vi "LoadTSConfigFile.vi"(0 "Sequence path":path=path "C:/ModisEdge/Scanner/Test Sequence/ModisEdgeScanner.ini", 5 "file name":string="ModisEdgeScanner.ini", 11 "error in (no error)":errorcluster) -> (2 "PS1_COMPort":string, 3 "InterlockDevice":string="Dev6", 4 "SnapOnTestScriptFile":string="G16_PD_TS_v3__G16_OC_TS_v2.txt", 6 "UUT_COMPort":string, 8 "DMM_COMPort":string, 10 "ResultsFolder":string="C:\\temp\\", 13 "PS2_COMPort":string, 14 "DAQDevice":string="Dev4", 15 "error out":errorcluster)   [LabVIEW 2015]
doc: "Use this template to build a VI to use as a subVI."
uses:
  <vilib>/Utility/config.llb/Read Key (String).vi
  <vilib>/Utility/config.llb/NI_LVConfig.lvlib
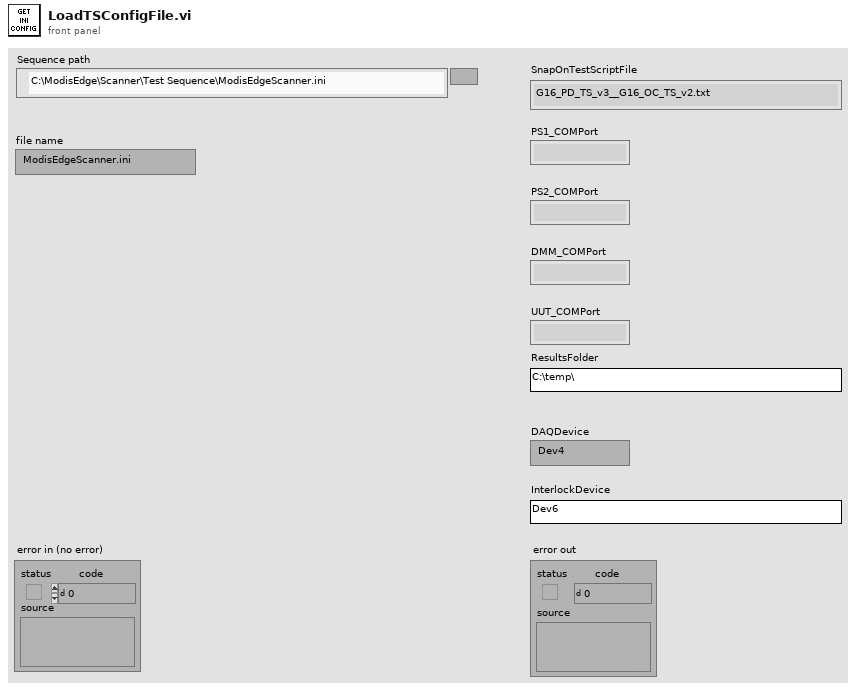
[diagram p1: front panel]
types:
  T1 = typedef "NI_LVConfig.lvlib/Config Data RefNum.ctl" = refnum<k1>
  T2 = typedef "Resource Data.ctl" = cluster{"Resource":string, "Serial Number":string, "Model":string}
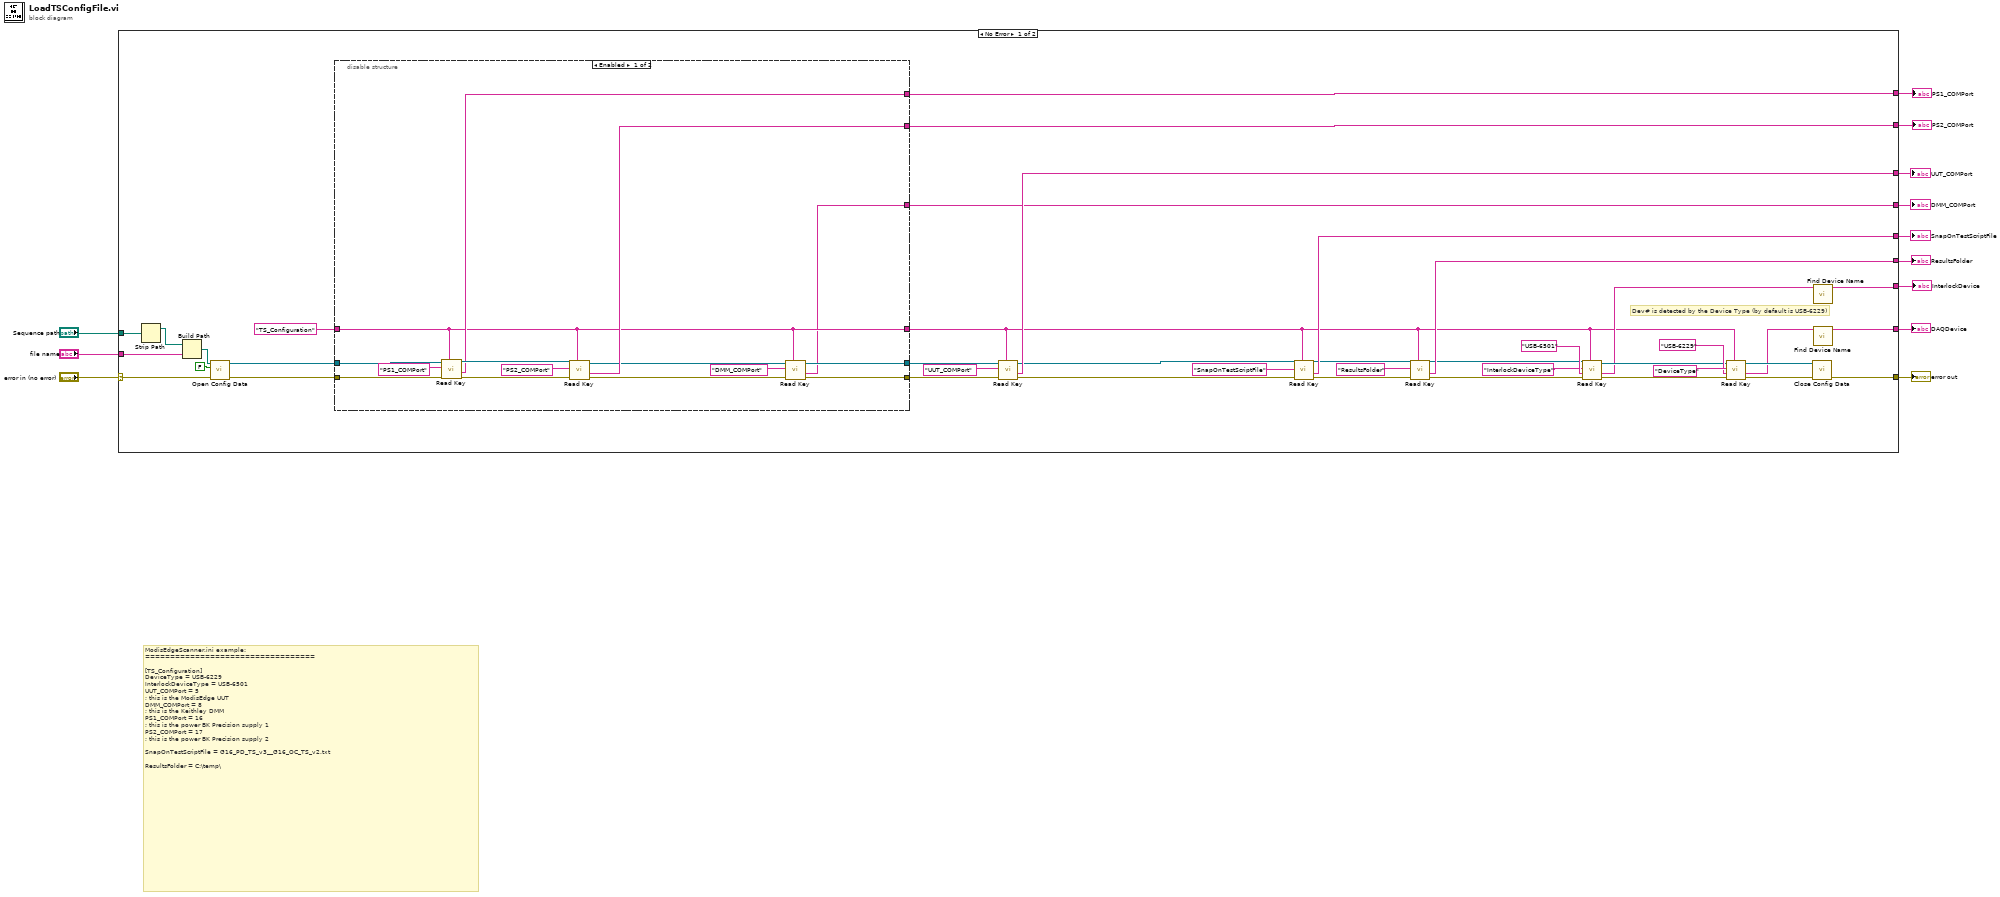
[diagram p0: block diagram]
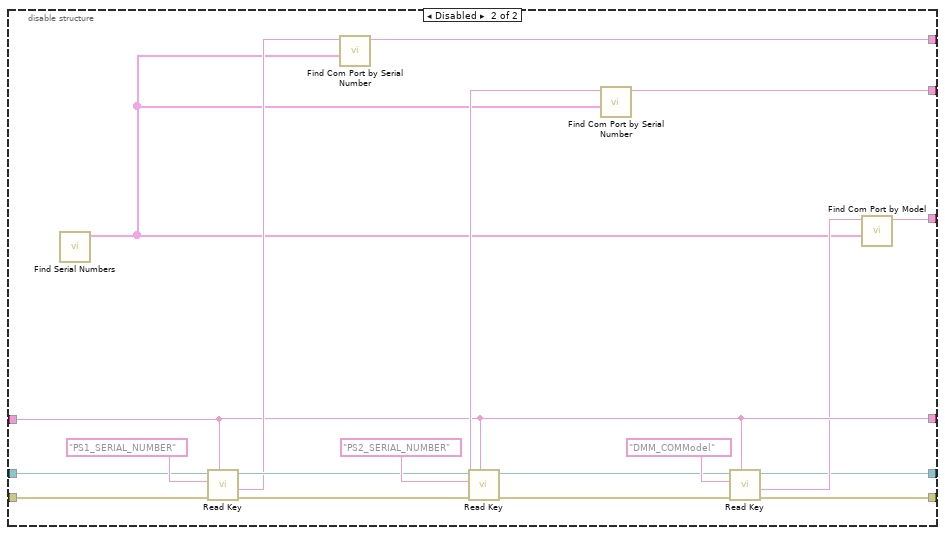
[diagram p2: hidden frame]
diagram:
  # "ModisEdgeScanner.ini example:\n==================================\n\n[TS_Configuration]\nDeviceType = USB-6229\nInterlockDeviceType = USB-6501\nUUT_COMPort = 5 \t\n; this is the ModisEdge UUT\nDMM_COMPort = 8\t\t\n; this is the Keithley DMM\nPS1_COMPort = 16\t\n; this is the power BK Precision supply 1 \nPS2_COMPort = 17\n; this is the power BK Precision supply 2\n\nSnapOnTestScriptFile = G16_PD_TS_v3__G16_OC_TS_v2.txt\n\nResultsFolder = C:\\temp\\"
  n1 = case shown="No Error" "error in (no error)" {
    selector: "error in (no error)" -> [w49 w87]
    tunnel: [w47 w87] -> w11
    tunnel: [w50 _] -> w10
    tunnel: [w48 _] -> w9
    tunnel: [w43 _] -> w8
    tunnel: "Sequence path" -> [w41 _]
    tunnel: [w35 _] -> w7
    tunnel: [w27 _] -> w6
    tunnel: [w16 _] -> w5
    tunnel: "file name" -> [w25 _]
    tunnel: [w22 _] -> w2
    tunnel: [w21 _] -> w1
    frame No Error {
      # "Dev# is detected by the Device Type (by default is USB-6229)"
      n2 = Strip Path(path=w41) -> (stripped path=w26:path)  [unwired: 1 out]
      n3 = Build Path(base path=w26, name or relative path=w25) -> (appended path=w42:path)
      n4 = call <vilib>:"Open Config Data.vi"("error in (no error)"=w49, "create file if necessary (T)"=FALSE, "configuration file path"=w42) -> ("error out"=w23:errorcluster, "refnum"=w20:T1)  [unwired: 6 in, 1 out]
      n5 = disable-structure shown="Enabled" {
        disable-tunnel: w23 -> [w63 w82]
        disable-tunnel: [w62 w80] -> w22
        disable-tunnel: [w61 w79] -> w21
        disable-tunnel: w20 -> [w60 w81]
        disable-tunnel: [w55 w74] -> w19
        disable-tunnel: [w54 w68] -> w18
        disable-tunnel: "TS_Configuration" ("key") -> [w56 w72]
        disable-tunnel: [w56 w72] -> w13
        disable-tunnel: [w53 w69] -> w16
        frame Enabled {
          n6 = call-poly <vilib>:"Read Key.vi"("section"=w56, "error in (no error)"=w63, "key"="PS1_COMPort", "refnum"=w60) -> ("error out"=w67:errorcluster, "value"=w62:string, "refnum out"=w66:T1)  [unwired: 4 in, 1 out]
          n7 = call-poly <vilib>:"Read Key.vi"("section"=w56, "error in (no error)"=w67, "key"="PS2_COMPort", "refnum"=w66) -> ("error out"=w58:errorcluster, "value"=w61:string, "refnum out"=w57:T1)  [unwired: 4 in, 1 out]
          n8 = call-poly <vilib>:"Read Key.vi"("section"=w56, "error in (no error)"=w58, "key"="DMM_COMPort", "refnum"=w57) -> ("error out"=w55:errorcluster, "value"=w53:string, "refnum out"=w54:T1)  [unwired: 4 in, 1 out]
        }
        frame Disabled {
          n9 = call "Find Serial Numbers.vi"() -> ("Array"=w70:T2[])  [unwired: 11 in]
          n10 = call-poly <vilib>:"Read Key.vi"("section"=w72, "error in (no error)"=w82, "key"="PS1_SERIAL_NUMBER", "refnum"=w81) -> ("error out"=w83:errorcluster, "value"=w78:string, "refnum out"=w84:T1)  [unwired: 4 in, 1 out]
          n11 = call "Find Com Port by Serial Number.vi"("Array"=w70, "Power Supply Serial Number"=w78) -> ("String"=w80:string)  [unwired: 9 in]
          n12 = call-poly <vilib>:"Read Key.vi"("section"=w72, "error in (no error)"=w83, "key"="PS2_SERIAL_NUMBER", "refnum"=w84) -> ("error out"=w75:errorcluster, "value"=w77:string, "refnum out"=w73:T1)  [unwired: 4 in, 1 out]
          n13 = call "Find Com Port by Serial Number.vi"("Array"=w70, "Power Supply Serial Number"=w77) -> ("String"=w79:string)  [unwired: 9 in]
          n14 = call-poly <vilib>:"Read Key.vi"("section"=w72, "error in (no error)"=w75, "key"="DMM_COMModel", "refnum"=w73) -> ("error out"=w74:errorcluster, "value"=w71:string, "refnum out"=w68:T1)  [unwired: 4 in, 1 out]
          n15 = call "Find Com Port by Model.vi"("Array"=w70, "Power Supply Serial Number"=w71) -> ("String"=w69:string)  [unwired: 9 in]
        }
      }
      n16 = call-poly <vilib>:"Read Key.vi"("section"=w13, "error in (no error)"=w19, "key"="UUT_COMPort", "refnum"=w18) -> ("error out"=w15:errorcluster, "value"=w48:string, "refnum out"=w14:T1)  [unwired: 4 in, 1 out]
      n17 = call-poly <vilib>:"Read Key.vi"("section"=w13, "error in (no error)"=w15, "key"="SnapOnTestScriptFile", "refnum"=w14) -> ("error out"=w44:errorcluster, "value"=w50:string, "refnum out"=w45:T1)  [unwired: 4 in, 1 out]
      n18 = call-poly <vilib>:"Read Key.vi"("section"=w13, "error in (no error)"=w44, "key"="ResultsFolder", "refnum"=w45) -> ("error out"=w32:errorcluster, "value"=w43:string, "refnum out"=w30:T1)  [unwired: 4 in, 1 out]
      n19 = call-poly <vilib>:"Read Key.vi"("section"=w13, "error in (no error)"=w32, "default value"="USB-6501", "key"="InterlockDeviceType", "refnum"=w30) -> ("error out"=w31:errorcluster, "value"=w28:string, "refnum out"=w29:T1)  [unwired: 3 in, 1 out]
      n20 = call-poly <vilib>:"Read Key.vi"("section"=w13, "error in (no error)"=w31, "default value"="USB-6229", "key"="DeviceType", "refnum"=w29) -> ("error out"=w39:errorcluster, "value"=w36:string, "refnum out"=w38:T1)  [unwired: 3 in, 1 out]
      n21 = call <vilib>:"Close Config Data.vi"("error in (no error)"=w39, "refnum"=w38) -> ("error out"=w47:errorcluster)  [unwired: 8 in, 1 out]
      n22 = call "Find Device Name.vi"("Device Type"=w28) -> ("Device Name"=w27:string)  [unwired: 10 in]
      n23 = call "Find Device Name.vi"("Device Type"=w36) -> ("Device Name"=w35:string)  [unwired: 10 in]
    }
    frame Error {
    }
  }
  "error out" <- w11
  "SnapOnTestScriptFile" <- w10
  "UUT_COMPort" <- w9
  "ResultsFolder" <- w8
  "DAQDevice" <- w7
  "InterlockDevice" <- w6
  "DMM_COMPort" <- w5
  "PS1_COMPort" <- w2
  "PS2_COMPort" <- w1
